vi "ElevatorExecuteLogic.vi"(6 "OuterPositionHeight":dbl, 7 "InnerPositionHeight":dbl, 8 "OuterLowLimitSwitch":bool, 9 "OuterHighLimitSwitch":bool, 10 "Stage3LowLimitSwitch":bool, 11 "Stage3HighLimitSwitch":bool) -> (1 "OuterMotorDemand":dbl, 3 "Stage3MotorDemand":dbl)   [LabVIEW 2023]
doc: "Holds the \"insides\" for the elevator execution"
uses:
  ElevatorSetpointEnum.ctl
  <vilib>/Rock Robotics/WPI/ThirdParty/JAS_Junk/TrajLib/VI/BoolCmd_Recv_Internal.vi
  <vilib>/Rock Robotics/WPI/ThirdParty/JAS_Junk/TrajLib/VI/BoolCmd_ObtainQueue.vi
  ElevatorGlobal.vi
  <vilib>/Rock Robotics/WPI/ThirdParty/JAS_Junk/TrajLib/Trajectory_Library.lvlib
panel:
  out "error out":errorcluster
  in  "error in (no error)":errorcluster
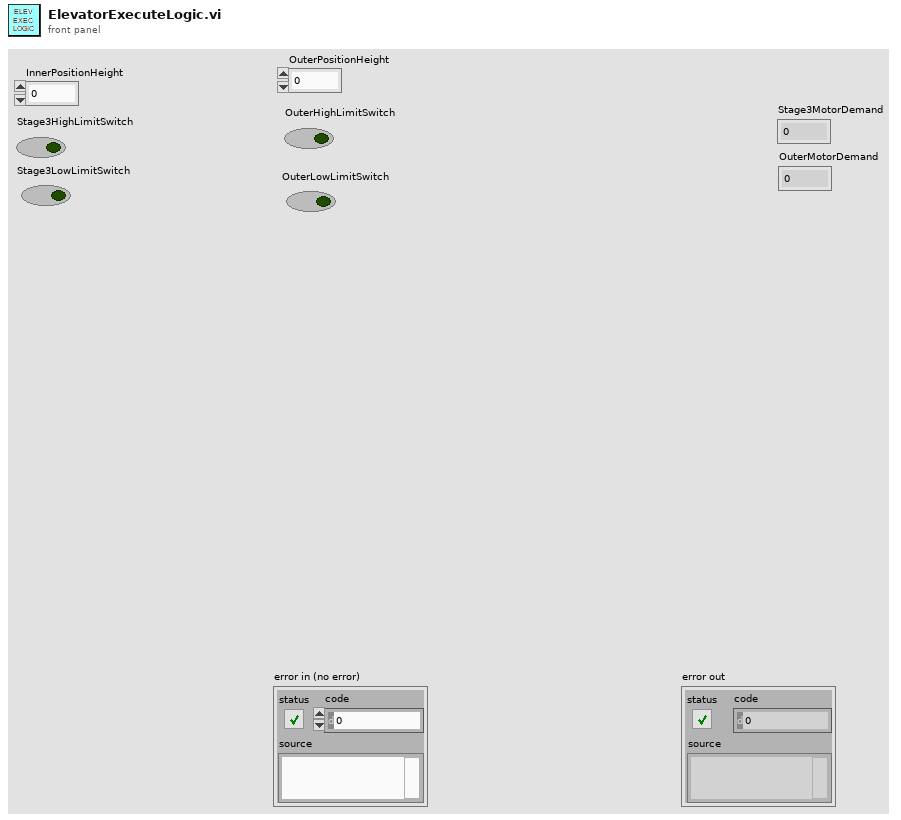
[diagram p1: front panel]
types:
  T1 = typedef "ElevatorSetpointEnum.ctl" = enum16{"Floor", "Rest", "Source", "L1", "L2", "Algae1", "L3", "Algae2", "L4", "Barge"}
  T2 = typedef "Trajectory_Library.lvlib/PosCtrl_Tuning_Type.ctl" = cluster{"Slope":dbl, "Offset":dbl, "Error Deadband":dbl, "At Reference Count":i32, "Negate Output":bool, "Max Allowd Position":dbl, "Min Allowd Position":dbl}
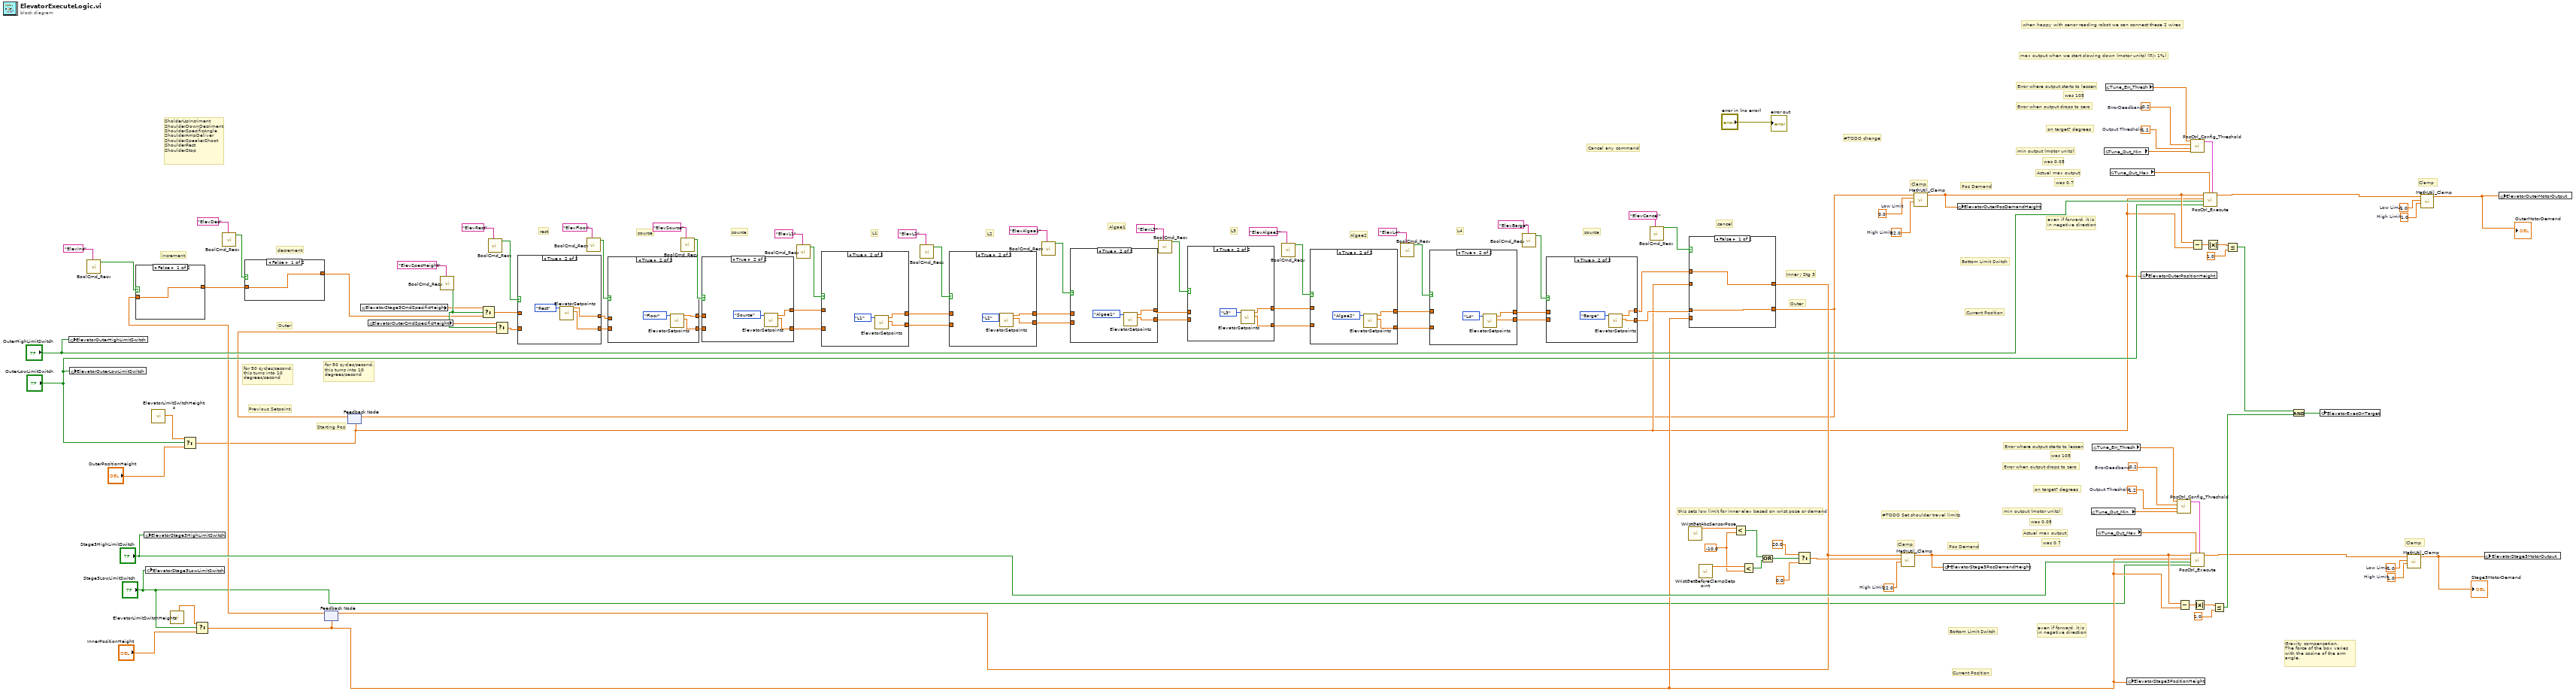
[diagram p0: block diagram]
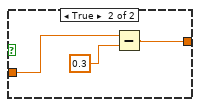
[diagram p4: hidden frame]
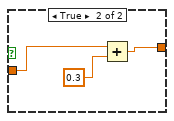
[diagram p5: hidden frame]
diagram:
  w24 = 0.0  # Low Limit
  w10 = -10.0 ("y")
  w61 = 22.0  # High Limit
  w63 = 1.0  # High Limit
  w62 = -1.0  # Low Limit
  w65 = 0.2  # ErrorDeadband
  w64 = 1.2  # Output Threshold
  w106 = 52.0  # High Limit
  w108 = 1.0  # High Limit
  w107 = -1.0  # Low Limit
  w111 = 0.2  # ErrorDeadband
  w110 = 1.2  # Output Threshold
  # "this sets low limit for inner elev based on wrist pose or demand"
  # "source"
  # "source"
  # "#TODO change"
  # "Outer"
  # "Inner / Stg 3"
  # "Outer"
  # "was 0.05"
  # "was 0.7"
  # "Actual max output"
  # "Current Position"
  # "Bottom Limit Switch"
  # "#TODO Set shoulder travel limits"
  # "Pos Demand"
  # "Clamp"
  # "was 105"
  # "Gravity compensation.\nThe force of the box varies\nwith the cosine of the arm\nangle."
  # "even if forward, it is \nin negative direction"
  # "Clamp"
  # "min output (motor units)"
  # "on target? degrees"
  # "Error when output drops to zero"
  # "Error where output starts to lessen"
  # "L4"
  # "Algae2"
  # "L3"
  # "Algae1"
  # "L2"
  # "L1"
  # "source"
  # "rest"
  # "SholderUpIncriment\nShoulderDownDecriment\nShoulderSpecificAngle\nShoulderAmpDeliver\nShoulderSpeakerShoot\nShoulderRest\nShoulderStop"
  # "was 0.05"
  # "was 0.7"
  # "Actual max output"
  # "Previous Setpoint."
  # "Current Position"
  # "Bottom Limit Switch"
  # "Starting Pos"
  # "for 50 cycles/second.\nthis turns into 10 \ndegrees/second"
  # "for 50 cycles/second.\nthis turns into 10 \ndegrees/second"
  # "increment"
  # "Pos Demand"
  # "Clamp"
  # "was 105"
  # "even if forward, it is \nin negative direction"
  # "Cancel any command"
  # "cancel"
  # "Clamp"
  # "decrement"
  # "when happy with senor reading robot we can connect these 2 wires"
  # "min output (motor units)"
  # "max output when we start slowing down (motor units) (=/- 1%)"
  # "on target? degrees"
  # "Error when output drops to zero"
  # "Error where output starts to lessen"
  n1 = global write "ElevatorGlobal.vi" "ElevatorOuterHighLimitSwitch"("OuterHighLimitSwitch") -> ()
  n2 = global write "ElevatorGlobal.vi" "ElevatorOuterLowLimitSwitch"("OuterLowLimitSwitch") -> ()
  n3 = call <vilib>:"BoolCmd_Recv.vi"("Command Name"="ElevInc") -> ("New Request"=w3:bool)  [unwired: 9 in, 1 out]
  n4 = global write "ElevatorGlobal.vi" "ElevatorStage3HighLimitSwitch"("Stage3HighLimitSwitch") -> ()
  n5 = global write "ElevatorGlobal.vi" "ElevatorStage3LowLimitSwitch"("Stage3LowLimitSwitch") -> ()
  n6 = call "ElevatorLimitSwitchHeights.vi"() -> ("LowOuter"=w82:dbl)  [unwired: 7 in, 4 out]
  n7 = call "ElevatorLimitSwitchHeights.vi"() -> ("LowStage3"=w41:dbl)  [unwired: 7 in, 4 out]
  n8 = Select(t=w82, s="OuterLowLimitSwitch", f="OuterPositionHeight") -> (s? t:f=w9:dbl)
  n9 = Select(t=w41, s="Stage3LowLimitSwitch", f="InnerPositionHeight") -> (s? t:f=w40:dbl)
  n10 = call <vilib>:"BoolCmd_Recv.vi"("Command Name"="ElevDec") -> ("New Request"=w1:bool)  [unwired: 9 in, 1 out]
  n11 = feedback #1(w40) -> (w35:dbl)
  n12 = case shown="False" w3 {
    tunnel: w35 -> [w113 w115]
    tunnel: [w113 w114] -> w34
    frame False {
    }
    frame True {
      n13 = Add(x=w115, y=0.3) -> (x+y=w114:dbl)
    }
  }
  n14 = case shown="False" w1 {
    tunnel: w34 -> [w117 w119]
    tunnel: [w117 w118] -> w33
    frame False {
    }
    frame True {
      n15 = Subtract(x=w119, y=0.3) -> (x-y=w118:dbl)
    }
  }
  n16 = feedback #2(w9) -> (w32:dbl)
  n17 = global read "ElevatorGlobal.vi" "ElevatorStage3CmdSpecificHeight"() -> (w30:dbl)
  n18 = global read "ElevatorGlobal.vi" "ElevatorOuterCmdSpecificHeight"() -> (w31:dbl)
  n19 = call <vilib>:"BoolCmd_Recv.vi"("Command Name"="ElevSpecHeight") -> ("New Request"=w38:bool)  [unwired: 9 in, 1 out]
  n20 = Select(t=w30, s=w38, f=w33) -> (s? t:f=w93:dbl)
  n21 = call <vilib>:"BoolCmd_Recv.vi"("Command Name"="ElevRest") -> ("New Request"=w102:bool)  [unwired: 9 in, 1 out]
  n22 = Select(t=w31, s=w38, f=w32) -> (s? t:f=w39:dbl)
  n23 = case shown="True" w102 {
    tunnel: w93 -> [w122 _]
    tunnel: [w122 w125] -> w21
    tunnel: [w121 w123] -> w20
    tunnel: w39 -> [w121 _]
    frame False {
    }
    frame True {
      n24 = call "ElevatorSetpoints.vi"("ElevatorSetpoints"=ElevatorSetpointEnum."Rest") -> ("OuterTargetHeight"=w123:dbl, "Stage3TargetHeight"=w125:dbl)  [unwired: 8 in, 1 out]
    }
  }
  n25 = call <vilib>:"BoolCmd_Recv.vi"("Command Name"="ElevFloor") -> ("New Request"=w23:bool)  [unwired: 9 in, 1 out]
  n26 = case shown="True" w23 {
    tunnel: [w127 w130] -> w19
    tunnel: [w126 w128] -> w18
    tunnel: w21 -> [w127 _]
    tunnel: w20 -> [w126 _]
    frame False {
    }
    frame True {
      n27 = call "ElevatorSetpoints.vi"("ElevatorSetpoints"=ElevatorSetpointEnum."Floor") -> ("OuterTargetHeight"=w128:dbl, "Stage3TargetHeight"=w130:dbl)  [unwired: 8 in, 1 out]
    }
  }
  n28 = call <vilib>:"BoolCmd_Recv.vi"("Command Name"="ElevSource") -> ("New Request"=w103:bool)  [unwired: 9 in, 1 out]
  n29 = case shown="True" w103 {
    tunnel: w19 -> [w132 _]
    tunnel: [w132 w135] -> w105
    tunnel: [w131 w133] -> w48
    tunnel: w18 -> [w131 _]
    frame False {
    }
    frame True {
      n30 = call "ElevatorSetpoints.vi"("ElevatorSetpoints"=ElevatorSetpointEnum."Source") -> ("OuterTargetHeight"=w133:dbl, "Stage3TargetHeight"=w135:dbl)  [unwired: 8 in, 1 out]
    }
  }
  n31 = call <vilib>:"BoolCmd_Recv.vi"("Command Name"="ElevL1") -> ("New Request"=w104:bool)  [unwired: 9 in, 1 out]
  n32 = case shown="True" w104 {
    tunnel: w105 -> [w137 _]
    tunnel: [w137 w140] -> w92
    tunnel: [w136 w138] -> w49
    tunnel: w48 -> [w136 _]
    frame False {
    }
    frame True {
      n33 = call "ElevatorSetpoints.vi"("ElevatorSetpoints"=ElevatorSetpointEnum."L1") -> ("OuterTargetHeight"=w138:dbl, "Stage3TargetHeight"=w140:dbl)  [unwired: 8 in, 1 out]
    }
  }
  n34 = call <vilib>:"BoolCmd_Recv.vi"("Command Name"="ElevL2") -> ("New Request"=w87:bool)  [unwired: 9 in, 1 out]
  n35 = case shown="True" w87 {
    tunnel: [w142 w145] -> w91
    tunnel: w92 -> [w142 _]
    tunnel: [w141 w143] -> w50
    tunnel: w49 -> [w141 _]
    frame False {
    }
    frame True {
      n36 = call "ElevatorSetpoints.vi"("ElevatorSetpoints"=ElevatorSetpointEnum."L2") -> ("OuterTargetHeight"=w143:dbl, "Stage3TargetHeight"=w145:dbl)  [unwired: 8 in, 1 out]
    }
  }
  n37 = call <vilib>:"BoolCmd_Recv.vi"("Command Name"="ElevAlgae1") -> ("New Request"=w86:bool)  [unwired: 9 in, 1 out]
  n38 = case shown="True" w86 {
    tunnel: [w147 w150] -> w90
    tunnel: w91 -> [w147 _]
    tunnel: [w146 w148] -> w51
    tunnel: w50 -> [w146 _]
    frame False {
    }
    frame True {
      n39 = call "ElevatorSetpoints.vi"("ElevatorSetpoints"=ElevatorSetpointEnum."Algae1") -> ("OuterTargetHeight"=w148:dbl, "Stage3TargetHeight"=w150:dbl)  [unwired: 8 in, 1 out]
    }
  }
  n40 = call <vilib>:"BoolCmd_Recv.vi"("Command Name"="ElevL3") -> ("New Request"=w85:bool)  [unwired: 9 in, 1 out]
  n41 = case shown="True" w85 {
    tunnel: [w152 w155] -> w89
    tunnel: w90 -> [w152 _]
    tunnel: [w151 w153] -> w52
    tunnel: w51 -> [w151 _]
    frame False {
    }
    frame True {
      n42 = call "ElevatorSetpoints.vi"("ElevatorSetpoints"=ElevatorSetpointEnum."L3") -> ("OuterTargetHeight"=w153:dbl, "Stage3TargetHeight"=w155:dbl)  [unwired: 8 in, 1 out]
    }
  }
  n43 = call <vilib>:"BoolCmd_Recv.vi"("Command Name"="ElevAlgae2") -> ("New Request"=w84:bool)  [unwired: 9 in, 1 out]
  n44 = case shown="True" w84 {
    tunnel: w89 -> [w157 _]
    tunnel: [w157 w160] -> w88
    tunnel: [w156 w158] -> w53
    tunnel: w52 -> [w156 _]
    frame False {
    }
    frame True {
      n45 = call "ElevatorSetpoints.vi"("ElevatorSetpoints"=ElevatorSetpointEnum."Algae2") -> ("OuterTargetHeight"=w158:dbl, "Stage3TargetHeight"=w160:dbl)  [unwired: 8 in, 1 out]
    }
  }
  n46 = call <vilib>:"BoolCmd_Recv.vi"("Command Name"="ElevL4") -> ("New Request"=w83:bool)  [unwired: 9 in, 1 out]
  n47 = case shown="True" w83 {
    tunnel: [w162 w165] -> w13
    tunnel: w88 -> [w162 _]
    tunnel: [w161 w163] -> w15
    tunnel: w53 -> [w161 _]
    frame False {
    }
    frame True {
      n48 = call "ElevatorSetpoints.vi"("ElevatorSetpoints"=ElevatorSetpointEnum."L4") -> ("OuterTargetHeight"=w163:dbl, "Stage3TargetHeight"=w165:dbl)  [unwired: 8 in, 1 out]
    }
  }
  n49 = call <vilib>:"BoolCmd_Recv.vi"("Command Name"="ElevBarge") -> ("New Request"=w17:bool)  [unwired: 9 in, 1 out]
  n50 = case shown="True" w17 {
    tunnel: [w166 w170] -> w12
    tunnel: [w167 w168] -> w14
    tunnel: w15 -> [w167 _]
    tunnel: w13 -> [w166 _]
    frame False {
    }
    frame True {
      n51 = call "ElevatorSetpoints.vi"("ElevatorSetpoints"=ElevatorSetpointEnum."Barge") -> ("OuterTargetHeight"=w168:dbl, "Stage3TargetHeight"=w170:dbl)  [unwired: 8 in, 1 out]
    }
  }
  n52 = call <vilib>:"BoolCmd_Recv.vi"("Command Name"="ElevCancel") -> ("New Request"=w100:bool)  [unwired: 9 in, 1 out]
  n53 = call "WristGetAbsSensorPose.vi"() -> ("WristAbsSensor"=w26:dbl)  [unwired: 11 in]
  n54 = case shown="False" w100 {
    tunnel: w12 -> [w172 _]
    tunnel: [w172 w174] -> w29
    tunnel: w9 -> [_ w174]
    tunnel: [w171 w173] -> w8
    tunnel: w14 -> [w171 _]
    tunnel: w40 -> [_ w173]
    frame False {
    }
    frame True {
      # "----------------------------------"
      # "takes get sensor pose pose"
    }
  }
  n55 = feedback-in #1(w29) -> ()
  n56 = feedback-in #2(w8) -> ()
  n57 = call "WristGetBeforeClampSetpoint.vi"() -> ("WristGetBeforeClampSetpoint"=w11:dbl)  [unwired: 11 in]
  n58 = Less?(x=w26, y=w10) -> (x < y?=w5:bool)
  n59 = Less?(x=w11, y=w10) -> (x < y?=w7:bool)
  n60 = Or(x=w5, y=w7) -> (x .or. y?=w6:bool)
  n61 = Select(t=20.0, s=w6, f=0.0) -> (s? t:f=w25:dbl)
  n62 = call <vilib>:"MathUtil_Clamp.vi"("High Limit"=w61, "Low Limit"=w25, "Value"=w29) -> ("Result"=w46:dbl)  [unwired: 8 in]
  n63 = call <vilib>:"MathUtil_Clamp.vi"("High Limit"=w106, "Low Limit"=w24, "Value"=w8) -> ("Result"=w70:dbl)  [unwired: 8 in]
  n64 = global write "ElevatorGlobal.vi" "ElevatorStage3PosDemandHeight"(w46) -> ()
  n65 = global write "ElevatorGlobal.vi" "ElevatorOuterPosDemandHeight"(w70) -> ()
  n66 = global read "ElevatorGlobal.vi" "Tune_Out_Min"() -> (w56:dbl)
  n67 = global read "ElevatorGlobal.vi" "Tune_Err_Thresh"() -> (w55:dbl)
  n68 = global read "ElevatorGlobal.vi" "Tune_Out_Max"() -> (w57:dbl)
  n69 = global read "ElevatorGlobal.vi" "Tune_Out_Min"() -> (w95:dbl)
  n70 = global read "ElevatorGlobal.vi" "Tune_Err_Thresh"() -> (w94:dbl)
  n71 = global read "ElevatorGlobal.vi" "Tune_Out_Max"() -> (w96:dbl)
  n72 = global write "ElevatorGlobal.vi" "ElevatorStage3PositionHeight"(w40) -> ()
  n73 = global write "ElevatorGlobal.vi" "ElevatorOuterPositionHeight"(w9) -> ()
  n74 = call <vilib>:"PosCtrl_Config_Threshold.vi"("Output Deadband"=w56, "Output Threshold"=w64, "ErrorDeadband"=w65, "ErrorThreshold"=w55) -> ("PosCtrl_Config_Params"=w66:T2)  [unwired: 7 in]
  n75 = Subtract(x=w46, y=w40) -> (x-y=w60:dbl)
  n76 = call <vilib>:"PosCtrl_Config_Threshold.vi"("Output Deadband"=w95, "Output Threshold"=w110, "ErrorDeadband"=w111, "ErrorThreshold"=w94) -> ("PosCtrl_Config_Params"=w112:T2)  [unwired: 7 in]
  n77 = call <vilib>:"PosCtrl_Execute.vi"("PosCtrl_Config_Params"=w66, "MaxOutput"=w57, "Rev Limit Switch"="Stage3LowLimitSwitch", "Fwd Limit Switch"="Stage3HighLimitSwitch", "CurrentPosition"=w40, "TargetPosition"=w46) -> ("Output"=w37:dbl)  [unwired: 3 in, 2 out]
  n78 = Subtract(x=w70, y=w9) -> (x-y=w99:dbl)
  n79 = Absolute Value(x=w60) -> (abs(x)=w59:dbl)
  n80 = call <vilib>:"PosCtrl_Execute.vi"("PosCtrl_Config_Params"=w112, "MaxOutput"=w96, "Rev Limit Switch"="OuterLowLimitSwitch", "Fwd Limit Switch"="OuterHighLimitSwitch", "CurrentPosition"=w9, "TargetPosition"=w70) -> ("Output"=w36:dbl)  [unwired: 3 in, 2 out]
  n81 = Absolute Value(x=w99) -> (abs(x)=w98:dbl)
  n82 = Less Or Equal?(x=w59, y=1.0) -> (x <= y?=w43:bool)
  n83 = Less Or Equal?(x=w98, y=1.0) -> (x <= y?=w42:bool)
  n84 = And(x=w42, y=w43) -> (x .and. y?=w44:bool)
  n85 = global write "ElevatorGlobal.vi" "ElevatorExecOnTarget"(w44) -> ()
  n86 = call <vilib>:"MathUtil_Clamp.vi"("High Limit"=w63, "Low Limit"=w62, "Value"=w37) -> ("Result"=w54:dbl)  [unwired: 8 in]
  "Stage3MotorDemand" <- w54
  n87 = call <vilib>:"MathUtil_Clamp.vi"("High Limit"=w108, "Low Limit"=w107, "Value"=w36) -> ("Result"=w69:dbl)  [unwired: 8 in]
  "OuterMotorDemand" <- w69
  n88 = global write "ElevatorGlobal.vi" "ElevatorStage3MotorOutput"(w54) -> ()
  n89 = global write "ElevatorGlobal.vi" "ElevatorOuterMotorOutput"(w69) -> ()
  "error out" <- "error in (no error)"
